vi "Check Array Term Type.vi"(7 "Dimensions Required":i32, 8 "error in (no error)":errorcluster, 9 "Element Check":T2, 10 "Dimension Check":T1, 11 "Term Type":T3) -> (0 "error out":errorcluster, 1 "Array Dimensions":i32, 2 "Element Type":variant, 3 "Is Good ?":bool)   [LabVIEW 2012, in "Scripting Tools.lvlib" / "XNode Support.lvlib"]
uses:
  XNode Support.lvlib
  <vilib>/XNodeSupport/XNodeTermTypeIDPair.ctl
  <vilib>/XNodeSupport/XNodeType.ctl
  <vilib>/XNodeSupport/XNodeString.ctl
  TypeDefs/Array element Tests.ctl
  TypeDefs/Array Dimension Tests.ctl
  <vilib>/Utility/VariantDataType/Type.ctl
  <vilib>/Utility/VariantDataType/VariantType.lvlib
  <vilib>/XNodeSupport/NI_XNodeSupport.lvlib
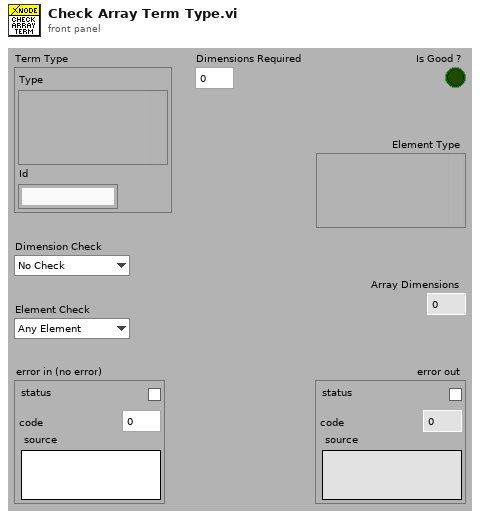
[diagram p1: front panel]
types:
  T1 = typedef "Scripting Tools.lvlib/XNode Support.lvlib/Array Dimension Tests.ctl" = enum16{"No Check", "At Least n dimensions", "Exactly N Dimensions", "No More Than N Dimensions"}
  T2 = typedef "Scripting Tools.lvlib/XNode Support.lvlib/Array element Tests.ctl" = enum16{"Any Element", "Numeric", "Integer", "Float", "Complex", "Boolean", "String", "Sortable"}
  T3 = typedef "NI_XNodeSupport.lvlib/XNodeTermTypeIDPair.ctl" = cluster{"Type":T4, "Id":T5}
  T4 = typedef "NI_XNodeSupport.lvlib/XNodeType.ctl" = variant
  T5 = typedef "NI_XNodeSupport.lvlib/XNodeString.ctl" = string
  T6 = typedef "VariantType.lvlib/Type.ctl" = enum8{"Invalid Type", "Void", "I8", "I16", "I32", "I64", "U8", "U16", "U32", "U64", "Single Float", "Double Float", "Extended Float", "Single Complex", "Double Complex", "Extended Complex", "Enum U8", "Enum U16", "Enum U32", "Enum U64", "Single Float With Unit", "Double Float With Unit", "Extended Float With Unit", "Single Complex with Unit", "Double Complex with Unit", "Extended Complex with Unit", "Boolean", "String", "Path", "Picture", "Tag", "Array", "Cluster", "Variant", "LV Variant", "Waveform", "Timestamp", "Digital Waveform", "Digital Data", "ExpressData", "Refnum", "External Data", "VI", "Poly VI", "LabVIEW Class Instance", "Fixed Point"}
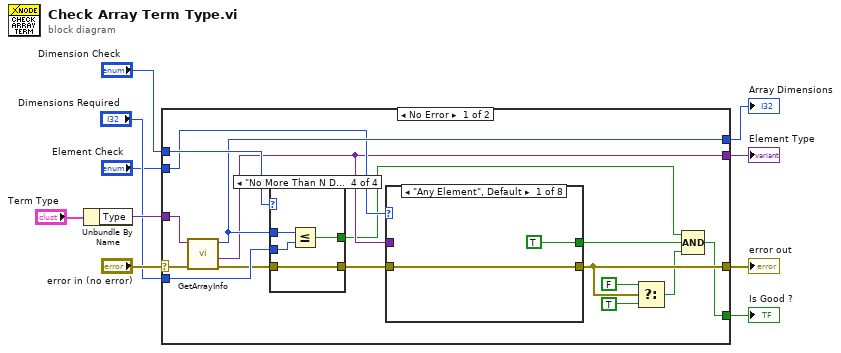
[diagram p0: block diagram]
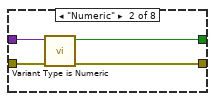
[diagram p2: hidden frame]
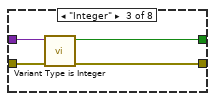
[diagram p3: hidden frame]
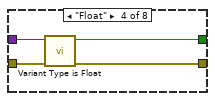
[diagram p4: hidden frame]
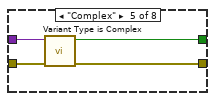
[diagram p5: hidden frame]
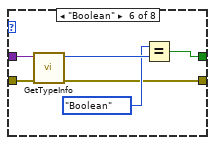
[diagram p6: hidden frame]
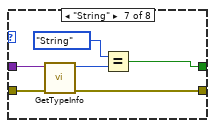
[diagram p7: hidden frame]
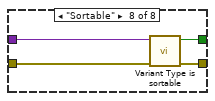
[diagram p8: hidden frame]
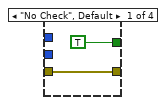
[diagram p9: hidden frame]
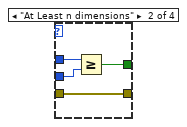
[diagram p10: hidden frame]
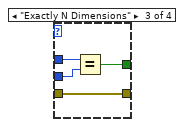
[diagram p11: hidden frame]
diagram:
  n1 = Unbundle By Name("Term Type") -> ("Type"=w8:T4)
  n2 = case shown="No Error" "error in (no error)" {
    selector: "error in (no error)" -> [w25 w75]
    tunnel: w8 -> [w26 _]
    tunnel: [w23 _] -> w7
    tunnel: [w18 _] -> w6
    tunnel: [w17 w75] -> w5
    tunnel: "Dimension Check" -> [w24 _]
    tunnel: "Dimensions Required" -> [w22 _]
    tunnel: "Element Check" -> [w21 _]
    tunnel: [w11 _] -> w1
    frame No Error {
      n3 = call <vilib>:"GetArrayInfo.vi"("error in (no error)"=w25, "Variant"=w26) -> ("error out"=w20:errorcluster, "ArrayElement"=w18:variant, "NDims"=w23:i32)  [unwired: 7 out]
      n4 = case shown="\"No More Than N Dimensions\"" w24 {
        tunnel: w23 -> [_ w66 w70 w74]
        tunnel: [TRUE w64 w68 w72] -> w12
        tunnel: w22 -> [_ w65 w69 w73]
        tunnel: w20 -> [w61 w63 w67 w71]
        tunnel: [w61 w63 w67 w71] -> w19
        frame "No Check", Default {
        }
        frame "At Least n dimensions" {
          n5 = Greater Or Equal?(x=w66, y=w65) -> (x >= y?=w64:bool)
        }
        frame "Exactly N Dimensions" {
          n6 = Equal?(x=w70, y=w69) -> (x = y?=w68:bool)
        }
        frame "No More Than N Dimensions" {
          n7 = Less Or Equal?(x=w74, y=w73) -> (x <= y?=w72:bool)
        }
      }
      n8 = case shown="\"Any Element\", Default" w21 {
        tunnel: [TRUE w29 w33 w37 w42 w46 w52 w58] -> w13
        tunnel: w19 -> [w27 w32 w35 w39 w44 w50 w56 w60]
        tunnel: [w27 w31 w34 w38 w41 w45 w51 w59] -> w17
        tunnel: w18 -> [_ w30 w36 w40 w43 w49 w55 w57]
        frame "Any Element", Default {
        }
        frame "Numeric" {
          n9 = call "Variant Type is Numeric.vi"("error in (no error)"=w32, "Type"=w30) -> ("error out"=w31:errorcluster, "Sortable ?"=w29:bool)  [unwired: 8 out]
        }
        frame "Integer" {
          n10 = call "Variant Type is Integer.vi"("error in (no error)"=w35, "Type"=w36) -> ("error out"=w34:errorcluster, "Sortable ?"=w33:bool)  [unwired: 8 out]
        }
        frame "Float" {
          n11 = call "Variant Type is Float.vi"("error in (no error)"=w39, "Type"=w40) -> ("error out"=w38:errorcluster, "Sortable ?"=w37:bool)  [unwired: 8 out]
        }
        frame "Complex" {
          n12 = call "Variant Type is Complex.vi"("error in (no error)"=w44, "Type"=w43) -> ("error out"=w41:errorcluster, "Sortable ?"=w42:bool)  [unwired: 8 out]
        }
        frame "Boolean" {
          n13 = call <vilib>:"GetTypeInfo.vi"("error in (no error)"=w50, "Variant"=w49) -> ("error out"=w45:errorcluster, "Type Enum"=w48:T6)  [unwired: 8 out]
          n14 = Equal?(x=Type."Boolean", y=w48) -> (x = y?=w46:bool)
        }
        frame "String" {
          n15 = call <vilib>:"GetTypeInfo.vi"("error in (no error)"=w56, "Variant"=w55) -> ("error out"=w51:errorcluster, "Type Enum"=w54:T6)  [unwired: 8 out]
          n16 = Equal?(x=Type."String", y=w54) -> (x = y?=w52:bool)
        }
        frame "Sortable" {
          n17 = call "Variant Type is sortable.vi"("error in (no error)"=w60, "Type"=w57) -> ("error out"=w59:errorcluster, "Sortable ?"=w58:bool)  [unwired: 8 out]
        }
      }
      n18 = Select(t=FALSE, s=w17, f=TRUE) -> (s? t:f=w14:bool)
      n19 = Compound Arithmetic op=AND(w12, w13, w14) -> (w11:bool)
    }
    frame Error {
    }
  }
  "error out" <- w5
  "Array Dimensions" <- w7
  "Element Type" <- w6
  "Is Good ?" <- w1
